vi "item select read.vi"(8 "error in (no error)":errorcluster, 11 "Listbox or Tree":refnum<vi>) -> (0 "error out":errorcluster, 1 "tags.disabled?":bool[](array[boolean]), 2 "tags.selected?":bool[](array[boolean]), 3 "tags.name":string[](array[string]), 5 "Tree":T1)   [LabVIEW 2020, in "UI_ItemSelect_OpenSource.lvlib"]
doc: "This method returns internall cached data pertaining to the status of selected states.\n\n<B>tags.name</B>\n<B>Listbox</B>: ItemNames\n<B>MCL</B>: First column of ItemNames\n<B>Tree</B>: Child-only tag names\n\n<B>selection states</B>\nTrue = item is selected\nArray length will always match array length of tags.name\n\n<B>selection locks</B>\nTrue = item is disabled and greyed out\nArray length will always match array length of tags.name\n\n<B>Tree</B>\nThis structure is only populated for Tree control references\nArray length = length of Tree.All tags\nThis structure is particularly useful for reading status of parent tree tags"
uses:
  UI_ItemSelect_OpenSource.lvlib
  SubVIs/Tree item loop data.ctl
  SubVIs/Tree item selection indices.ctl
  SubVIs/checkbox state.ctl
  SubVIs/item select tree lock states.ctl
  SubVIs/item select action.ctl
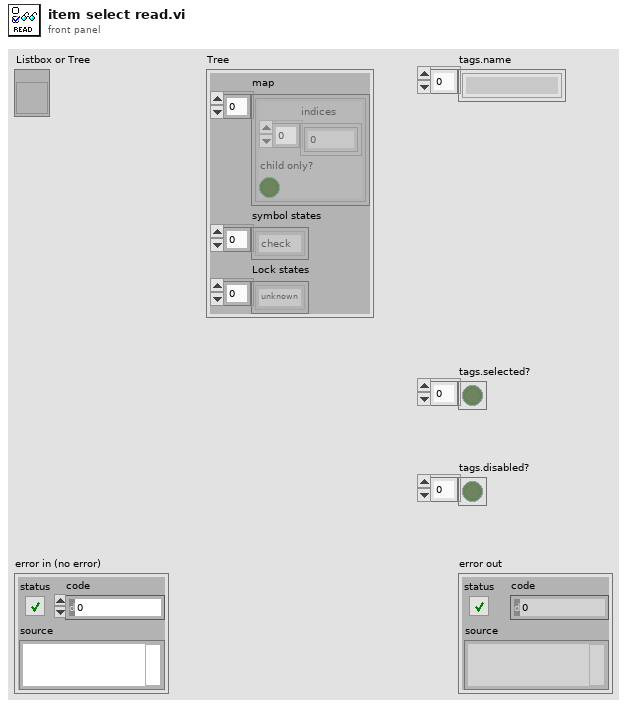
[diagram p1: front panel]
types:
  T1 = typedef "UI_ItemSelect_OpenSource.lvlib/Tree item loop data.ctl" = cluster{"map":T2[], "symbol states":T3[], "Lock states":T4[]}
  T2 = typedef "UI_ItemSelect_OpenSource.lvlib/Tree item selection indices.ctl" = cluster{"indices":i32[], "child only?":bool}
  T3 = typedef "UI_ItemSelect_OpenSource.lvlib/checkbox state.ctl" = enum16{"unknown", "check", "some", "no check"}
  T4 = typedef "UI_ItemSelect_OpenSource.lvlib/item select tree lock states.ctl" = enum16{"unknown", "locked", "unlocked"}
  T5 = typedef "UI_ItemSelect_OpenSource.lvlib/item select action.ctl" = enum16{"init", "read", "write states", "write locks", "mouse down", "delete", "select all", "select none", "invert selection"}
  T6 = typedef "UI_ItemSelect_OpenSource.lvlib/Tree item select loop data.ctl" = cluster{"Type":T7, "Ref":refnum<vi>, "LstBox Ref":refnum<vi>, "MCL Ref":refnum<vi>, "Tree Ref":refnum<vi>, "Last selected row":i32, "selection tags":string[], "selection states":bool[], "selection locks":bool[], "Tree":T1}
  T7 = typedef "UI_ItemSelect_OpenSource.lvlib/Item select ref type.ctl" = enum16{"Tree", "MCL", "ListBox"}
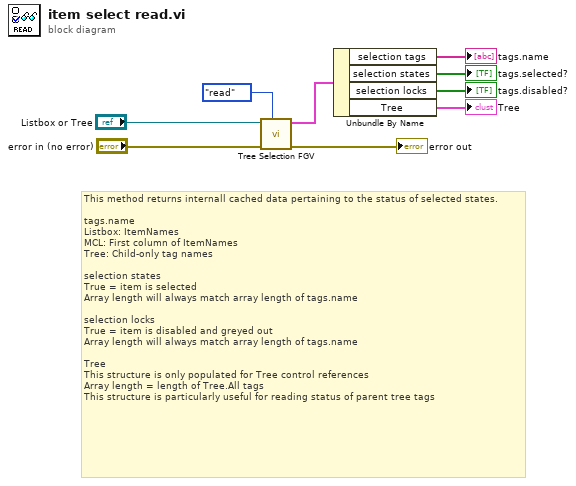
[diagram p0: block diagram]
diagram:
  # "This method returns internall cached data pertaining to the status of selected states.\n\ntags.name\nListbox: ItemNames\nMCL: First column of ItemNames\nTree: Child-only tag names\n\nselection states\nTrue = item is selected\nArray length will always match array length of tags.name\n\nselection locks\nTrue = item is disabled and greyed out\nArray length will always match array length of tags.name\n\nTree\nThis structure is only populated for Tree control references\nArray length = length of Tree.All tags\nThis structure is particularly useful for reading status of parent tree tags"
  n1 = call "Tree Selection FGV.vi"("Action"=item_select_action."read", "error in (no error)"="error in (no error)", "Listbox or Tree"="Listbox or Tree") -> ("error out"=→"error out":errorcluster, "read data"=w5:T6)  [unwired: 7 in]
  n2 = Unbundle By Name(w5) -> ("selection tags"=→"tags.name":string[], "selection states"=→"tags.selected?":bool[], "selection locks"=→"tags.disabled?":bool[], "Tree"=→"Tree":T1)
